vi "Write FPGA API.vi"(10 "FPGA API.lvclass":refnum<class "FPGA API.lvclass">, 11 "Device in":refnum<class "Device.lvclass">) -> (3 "Device out":refnum<class "Device.lvclass">)   [LabVIEW 2019, in "Device.lvclass"]
uses:
  Device.lvclass
  FPGA_API_class/FPGA API.lvclass
  Device.lvclass/Device.ctl
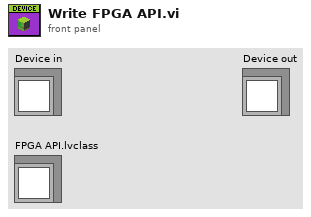
[diagram p1: front panel]
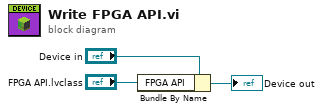
[diagram p0: block diagram]
diagram:
  n1 = Bundle By Name(cluster="Device in", "FPGA API"="FPGA API.lvclass") -> (→"Device out":refnum<class "Device.lvclass">)
